vi "Actor Core.vi"(8 "error in":errorcluster, 11 "Measure Object in":refnum<class "Spectrum Recorder too.lvclass">) -> (0 "error out":errorcluster, 3 "Actor out":refnum<class "Actor.lvclass">)   [LabVIEW 2016, in "Spectrum Recorder too.lvclass"]
doc: "(<B>Filename</B>: Actor Framework.lvlib:Actor.lvclass:Actor Core.vi)\n\nReceives messages to the actor, reacts to them, and initiates any error handling that may shut the actor down.\n\nDescendant classes may override this VI to append parallel tasks for the actor to complete while it handles messages. Overrides use the Call Parent Method node."
uses:
  Spectrum Recorder too.lvclass
  <vilib>/ActorFramework/Actor/Actor.lvclass
  NHMFL_Core/Libraries/Red Pitaya/RP Core/Red Pitaya Transceiver Driver/Spectrum Configuration.ctl
  Spectrum Recorder too.lvclass/Spectrum Recorder too.ctl
  Measure_core/Instrument Actor/Instrument Actor.lvclass
panel:
  out "Spectrum plot":cluster{dbl[], dbl[]}[](graph)
  in  "Configuration":T1={"Start"=500000.0, "End"=2000000.0, "Duration"=40.0, "Filter time constant"=0.004} {"Filter time constant" format="%#_6ps"; "Duration" format="%#_6ps"; "End" format="%#_6pHz"; "Start" format="%#_6pHz"}
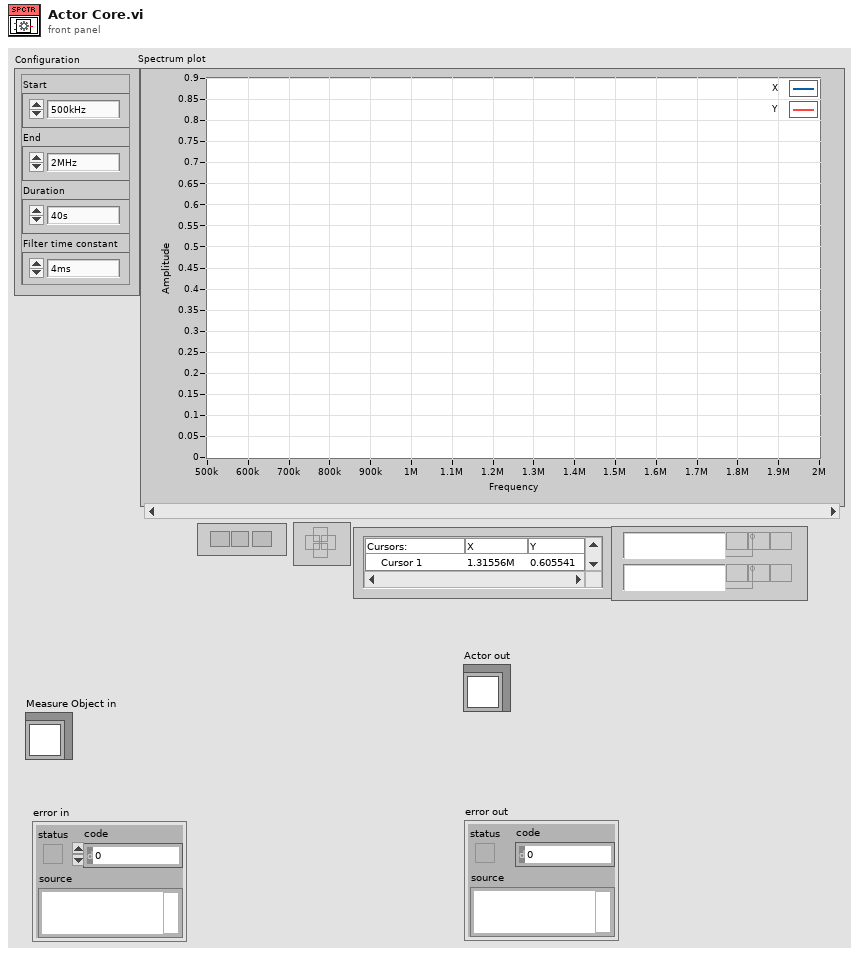
[diagram p1: front panel]
types:
  T1 = typedef "Spectrum Configuration.ctl" = cluster{"Start":dbl, "End":dbl, "Duration":dbl, "Filter time constant":dbl}
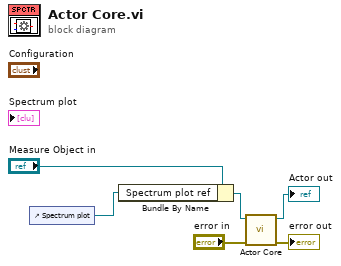
[diagram p0: block diagram]
diagram:
  n1 = control-ref of="Spectrum plot"() -> (w1:refnum<vi>)
  n2 = Bundle By Name(cluster="Measure Object in", "Spectrum plot ref"=w1) -> (w2:refnum<class "Spectrum Recorder too.lvclass">)
  n3 = call-parent "Actor Core.vi"("error in"="error in", "Measure Object in"=w2) -> ("error out"=→"error out":errorcluster, "Actor out"=→"Actor out":refnum<class "Actor.lvclass">)  [unwired: 8 in]
